vi "SigProc_subVI baselineRemoval.vi"(4 "Intervals":i32=200, 6 "Sub":dbl, 9 "Type":u8, 11 "waveform in":waveform(sgl)) -> (3 "waveform out":waveform(sgl))   [LabVIEW 2018, in "Sig2MS.lvclass"]
uses:
  Sig2MS.lvclass
  <vilib>/Analysis/baseanly.llb/Unimode.vi
  <vilib>/Analysis/NI_AALBase.lvlib
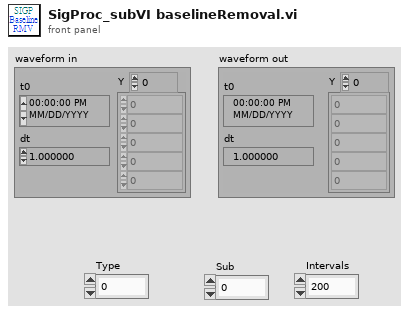
[diagram p1: front panel]
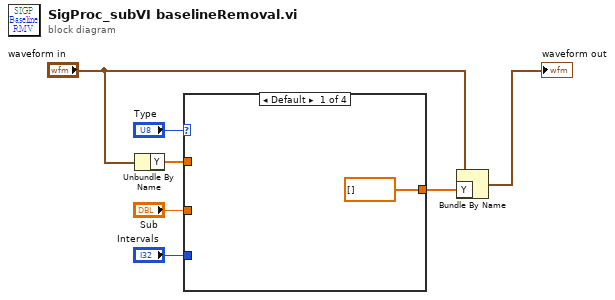
[diagram p0: block diagram]
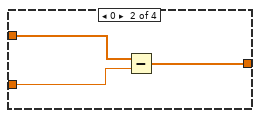
[diagram p2: hidden frame]
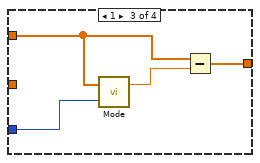
[diagram p3: hidden frame]
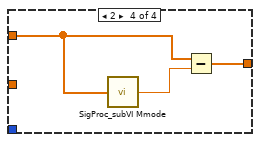
[diagram p4: hidden frame]
diagram:
  n1 = Unbundle By Name("waveform in") -> ("Y"=w1:sgl[])
  n2 = case shown="Default" "Type" {
    tunnel: w1 -> [_ w11 w15 w16]
    tunnel: "Sub" -> [_ w10 _ _]
    tunnel: [dbl[] [] w9 w13 w17] -> w3
    tunnel: "Intervals" -> [_ _ w12 _]
    frame Default {
    }
    frame 0 {
      n3 = Subtract(x=w11, y=w10) -> (x-y=w9:dbl[])
    }
    frame 1 {
      n4 = call-poly <vilib>:"Mode.vi"("intervals"=w12, "X"=w15) -> ("mode"=w14:dbl)  [unwired: 1 out]
      n5 = Subtract(x=w15, y=w14) -> (x-y=w13:dbl[])
    }
    frame 2 {
      n6 = call "SigProc_subVI Mmode.vi"("Y Data"=w16) -> ("element"=w18:dbl)
      n7 = Subtract(x=w16, y=w18) -> (x-y=w17:dbl[])
    }
  }
  n8 = Bundle By Name(cluster="waveform in", "Y"=w3) -> (→"waveform out":waveform(sgl))
